vi "Send.vi"(7 "LabVIEW Web Service Request":refnum<class "Web Request.lvclass">) -> ()   [LabVIEW 2016]
uses:
  <vilib>/wsapi/Web Request.lvclass
  AE Data.ctl
panel:
  out "error out":errorcluster
  # "Use the Web Service Request input terminal to call the VIs on the Web Services palette. Do not remove it from the connector pane unless you don't need access to the palette."
  # "Each additional control wired to the connector pane will be available as an input in the URL. To include an indicator in terminal-mode output (the default setting), it must also be wired to the connector pane."
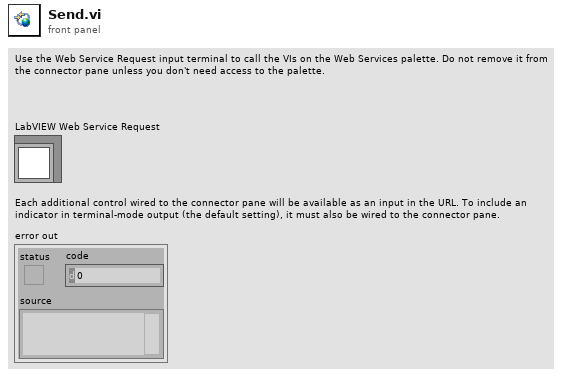
[diagram p1: front panel]
types:
  T1 = typedef "AE Data.ctl" = cluster{"Name":string, "Go?":bool, "Which batch?":enum16{"Anything", "First", "Second"}}
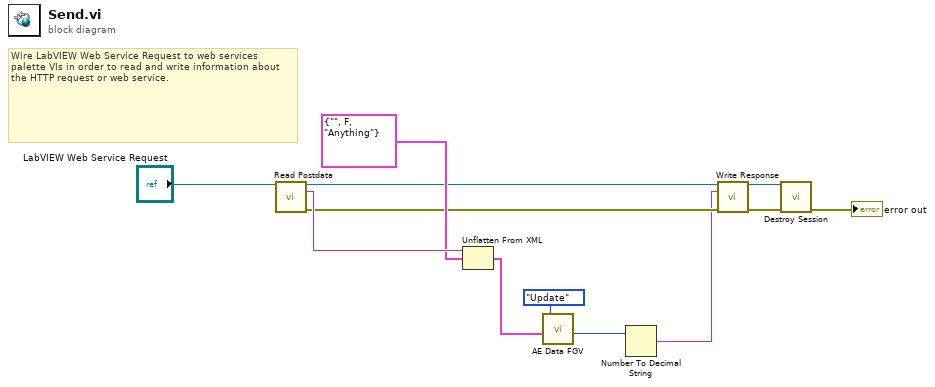
[diagram p0: block diagram]
diagram:
  # "Wire LabVIEW Web Service Request to web services palette VIs in order to read and write information about the HTTP request or web service."
  n1 = call <vilib>:"Read Postdata.vi"("LabVIEW Web Service Request"="LabVIEW Web Service Request") -> ("LabVIEW Web Service Request out"=w6:refnum<class "Web Request.lvclass">, "postdata"=w11:string, "error out"=w5:errorcluster)  [unwired: 12 in]
  n2 = Unflatten From XML(xml string=w11, type=T1 {"Name"="", "Go?"=FALSE, "Which batch?"=enum."Anything"} ("AE")) -> (value=w9:T1)  [unwired: 1 in, 1 out]
  n3 = call "AE Data FGV.vi"("AE"=w9, "Command"=enum16{"Initialize", "Update", "Get"}."Update") -> ("Index"=w7:i32)  [unwired: 8 in, 1 out]
  n4 = Number To Decimal String(number=w7) -> (decimal integer string=w4:string)  [unwired: 1 in]
  n5 = call <vilib>:"Write Response.vi"("LabVIEW Web Service Request"=w6, "response string"=w4, "error in (no error)"=w5) -> ("LabVIEW Web Service Request out"=w3:refnum<class "Web Request.lvclass">, "error out"=w2:errorcluster)  [unwired: 11 in]
  n6 = call <vilib>:"Destroy Session.vi"("LabVIEW Web Service Request"=w3, "error in (no error)"=w2) -> ("error out"=→"error out":errorcluster)  [unwired: 12 in, 1 out]
